vi "Log Errors.vi"(7 "section identifier":string, 10 "errors in":errorcluster[](array[cluster]), 11 "log file":path=path "c:/ni-rt/VeriStand/Custom Devices/Errors.txt") -> (0 "error out":errorcluster)   [LabVIEW 2020]
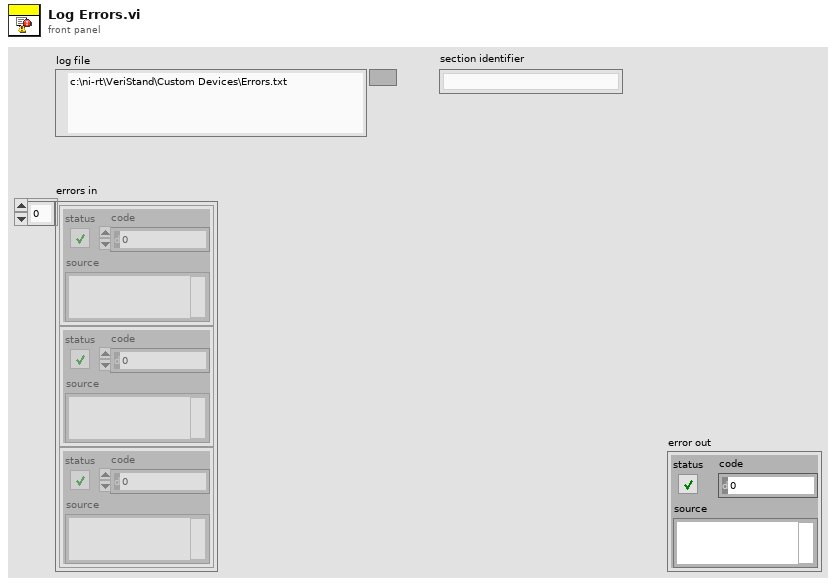
[diagram p1: front panel]
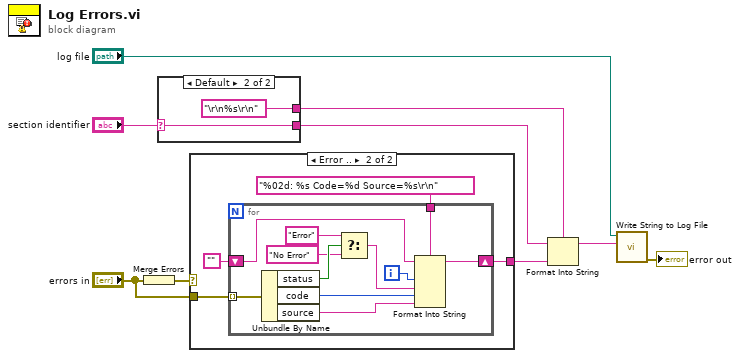
[diagram p0: block diagram]
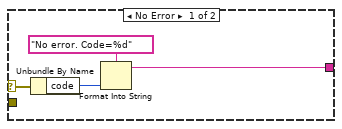
[diagram p2: hidden frame]
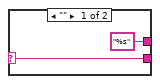
[diagram p3: hidden frame]
diagram:
  n1 = Merge Errors("errors in") -> (w8:errorcluster)
  n2 = case shown="Default" "section identifier" {
    selector: "section identifier" -> [w11 w12]
    tunnel: ["%s" ("format string") "\r\n%s\r\n" ("format string")] -> w6
    tunnel: [w11 w12] -> w2
    frame "" {
    }
    frame Default {
    }
  }
  n3 = case shown="Error .." w8 {
    selector: w8 -> [w17 _]
    tunnel: [w14 w20] -> w7
    tunnel: "errors in" -> [_ w21]
    frame No Error {
      n4 = Unbundle By Name(w17) -> ("code"=w16:i32)
      n5 = Format Into String(format string="No error. Code=%d", w16) -> (resulting string=w14:string)  [unwired: 2 in, 1 out]
    }
    frame Error {
      n6 = for {
        tunnel: w21 -> [w32] mode=indexing
        shift-right: [w24] -> w20
        shift-left: "" -> [w23]
        tunnel: "%02d: %s Code=%d Source=%s\r\n" ("format string") -> [w22]
        i -> [w25]
        n7 = Unbundle By Name(w32) -> ("status"=w31:bool, "code"=w27:i32, "source"=w26:string)
        n8 = Select(t="Error" ("source"), s=w31, f="No Error" ("source")) -> (s? t:f=w28:string)
        n9 = Format Into String(format string=w22, initial string=w23, w25, w28, w27, w26) -> (resulting string=w24:string)  [unwired: 1 in, 1 out]
      }
    }
  }
  n10 = Format Into String(format string=w6, initial string=w2, w7) -> (resulting string=w5:string)  [unwired: 1 in, 1 out]
  n11 = call "Write String to Log File.vi"("string to log"=w5, "log file"="log file") -> ("error out"=→"error out":errorcluster)  [unwired: 9 in]
